vi "LabVIEW Picture.vi"() -> ()   [LabVIEW 2012]
panel:
  out "DeviceIsOpen":bool
  out "Image":T1(plugin-control)
  out "Oil Value":sgl
  out "Water Value":sgl
  out "Output Picture 2":picture
  in  "Temporary File Path 2":path=path "E:/workforpetrol/Tem.bmp"
  in  "TempLate File 2":path=path "E:/workforpetrol/Temp/Template9.png"
  in  "Device Config File Path":path=path "E:/workforpetrol/image device.dat"
  in  "ICImagingControl":refnum<k7>(container)
  in  "Open Device Configuration (Monochrome  Images)":bool
  in  "End Program":bool
  # "Open Device Configuration"
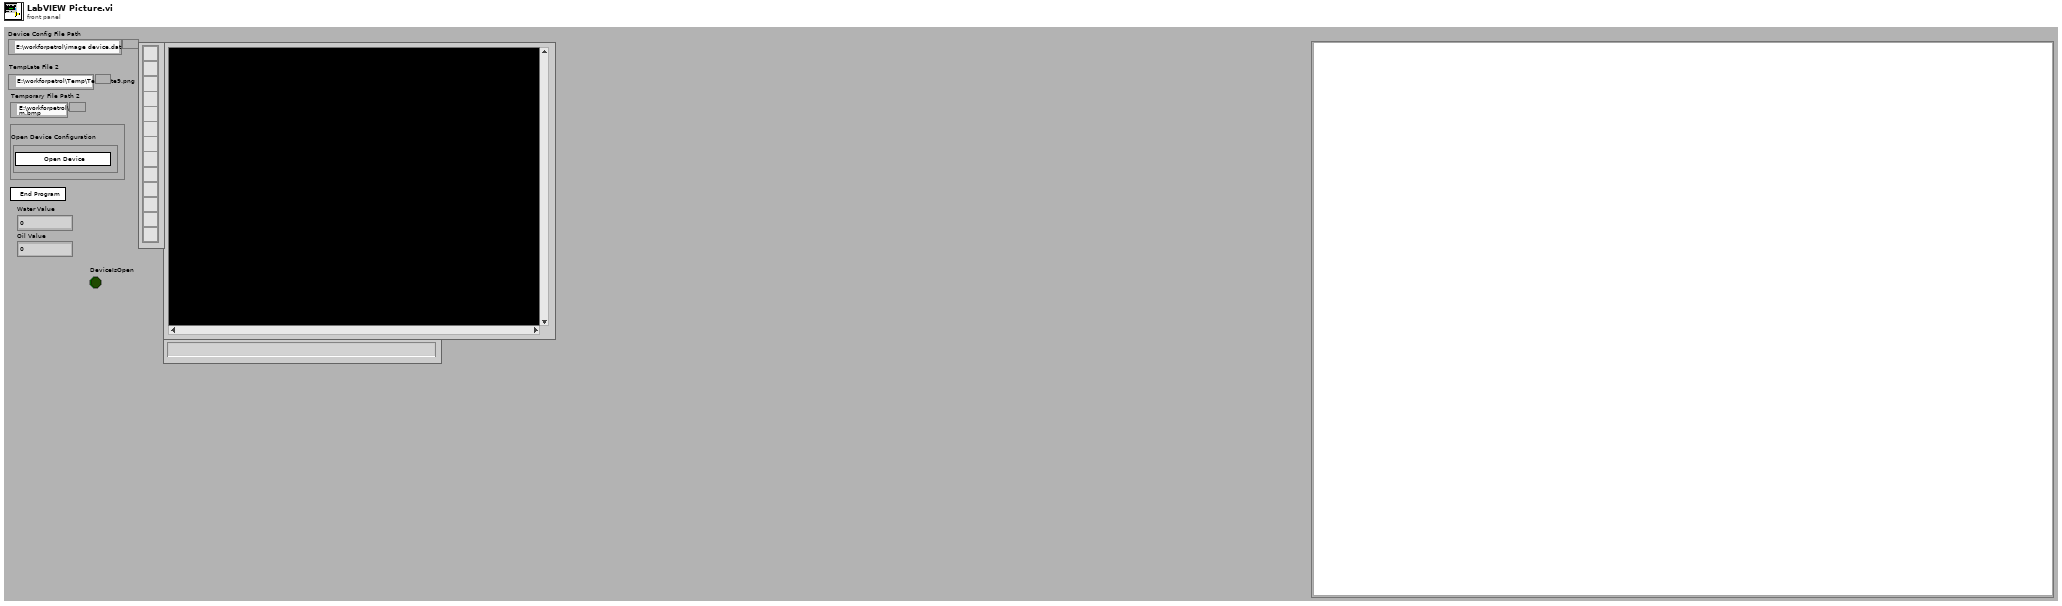
[diagram p1: front panel]
types:
  T1 = typedef "IMAQ Image.ctl" = refnum<image>
  T2 = typedef "imagedata.ctl" = cluster{"image type":i32, "image depth":i32, "image":u8[], "mask":u8[], "colors":u32[], "Rectangle":cluster{"left":i16, "top":i16, "right":i16, "bottom":i16}}
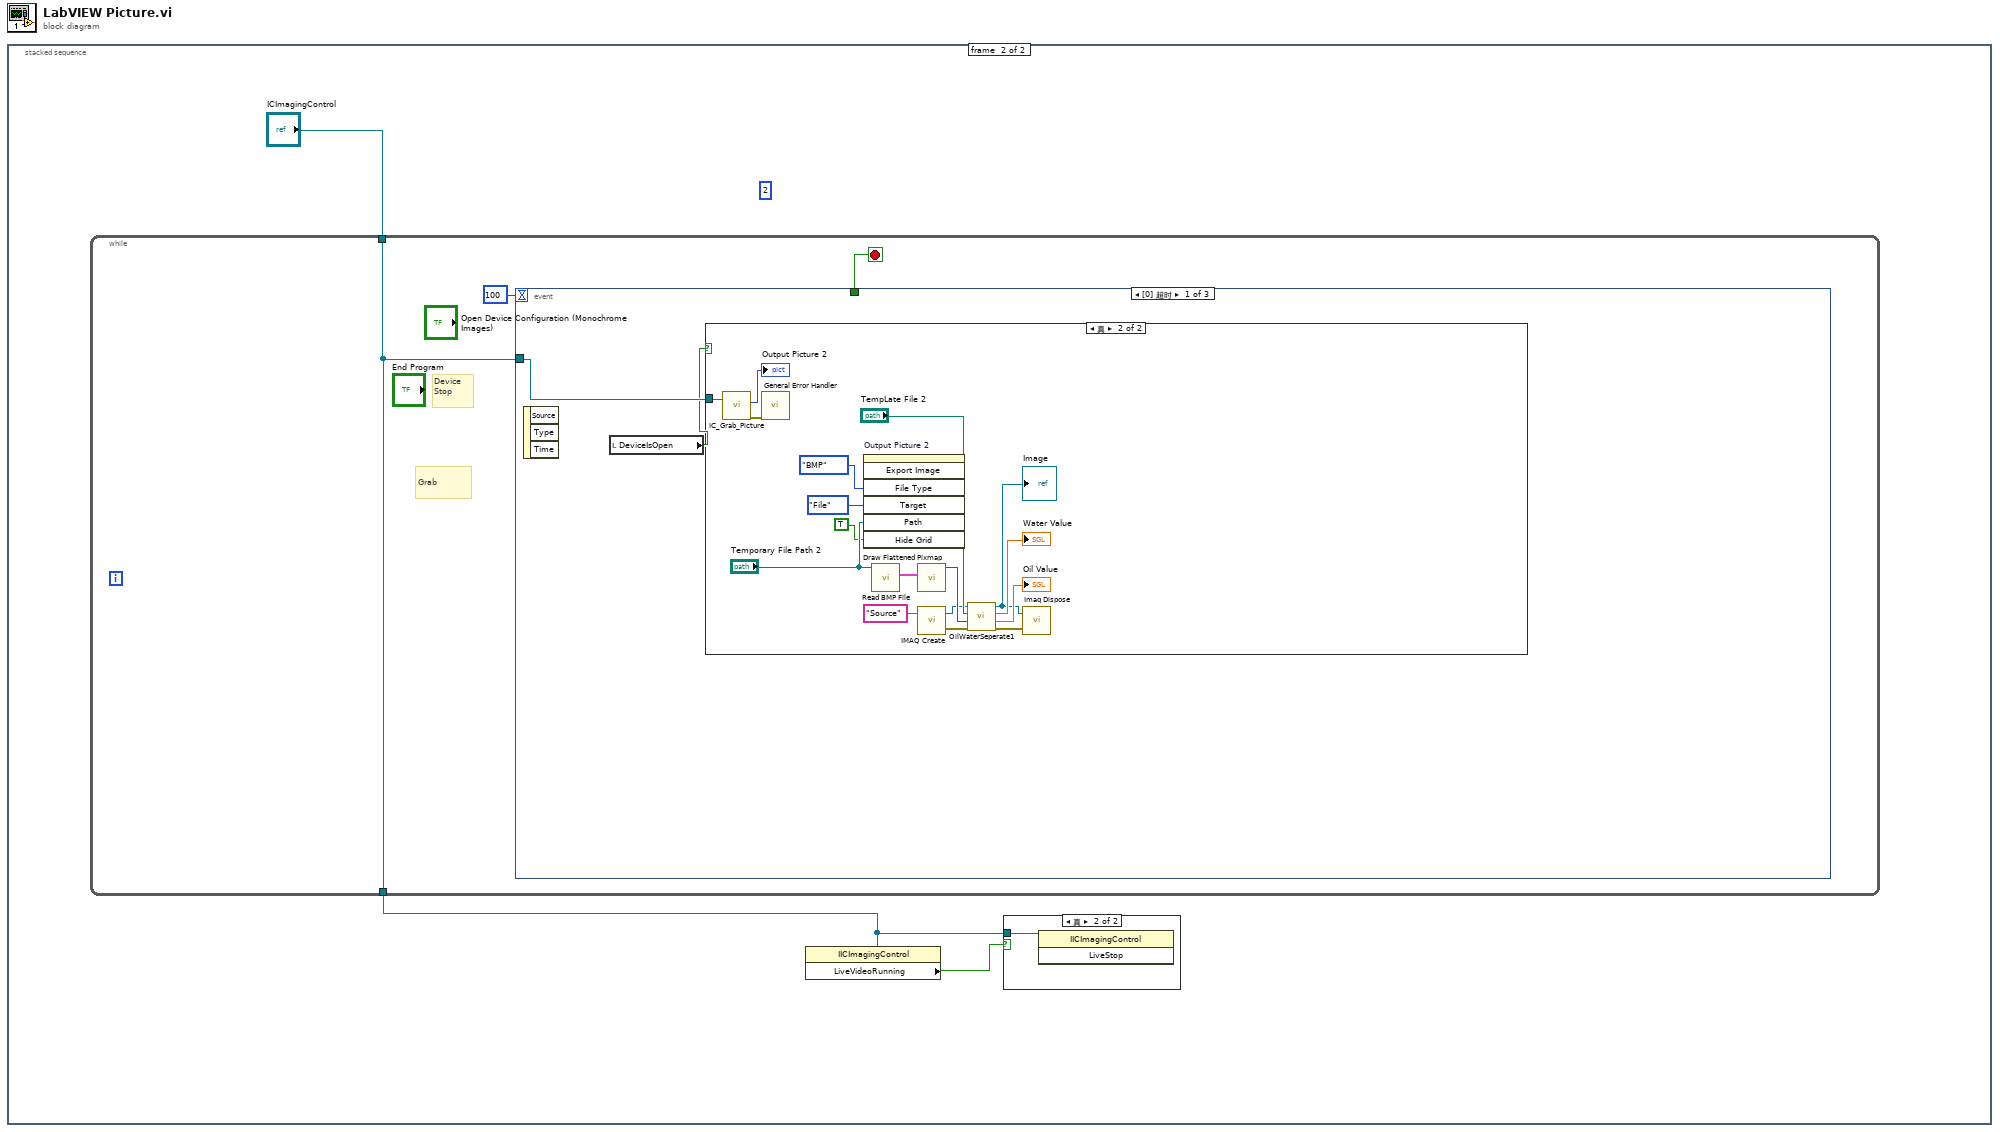
[diagram p0: block diagram]
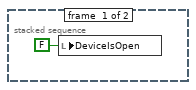
[diagram p2: hidden frame]
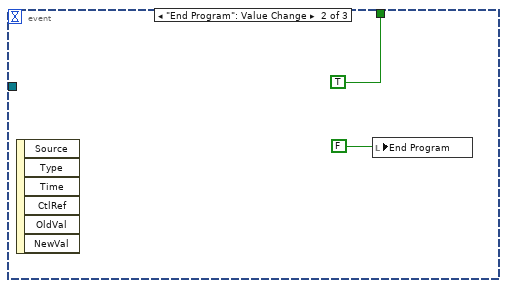
[diagram p5: hidden frame]
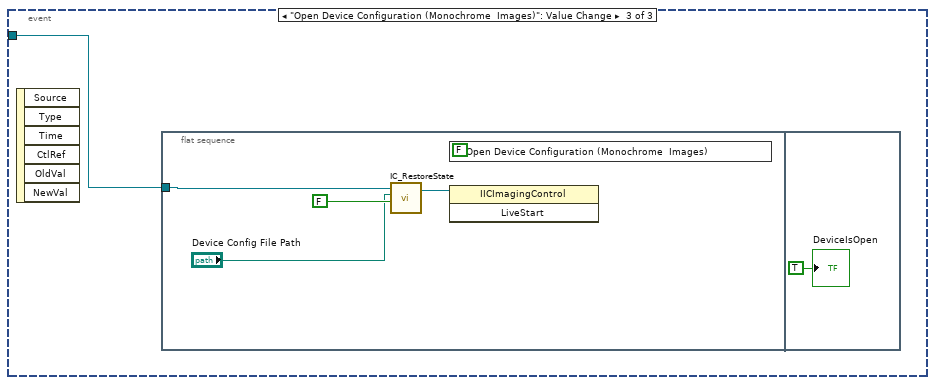
[diagram p6: hidden frame]
diagram:
  n1 = stacked-sequence {
    frame #0 {
      n2 = local write "DeviceIsOpen"(FALSE ("DeviceIsOpen")) -> ()
    }
    frame #1 {
      (unwired) u8 2 ("Disabled")
      n3 = while {
        tunnel: "ICImagingControl" -> [w7]
        tunnel: [w7] -> w3
        stop <- w8 stop-if-true
        # "Device\nStop"
        # "Grab"
        n4 = event shown="[0] 超时" {
          selector: _ -> [_ _ _]
          dyn-events: _ -> [_ _ _]
          timeout: 100 -> [_ _ _]
          tunnel: w7 -> [w10 _ w30]
          tunnel: [_ TRUE _] -> w8
          event Timeout {
            n5 = event-data() -> ()  [unwired: 1 in, 3 out]
            n6 = local read "DeviceIsOpen"() -> (w9:bool)
            n7 = case shown="真" w9 {
              tunnel: w10 -> [_ w25]
              frame False {
              }
              frame True {
                n8 = call "IC_Grab_Picture.vi"("ICImagingControl In"=w25) -> ("Picture Out"=→"Output Picture 2":picture, "Error Out"=w27:errorcluster)  [unwired: 1 in, 2 out]
                n9 = call <vilib>:"General Error Handler.vi"("error in (no error)"=w27) -> ()  [unwired: 10 in, 5 out]
                n10 = invoke on="Output Picture 2" class="Pict" method="Export Image"("File Type"=enum32{"BMP", "EPS", "EMF", "PICT"}."BMP" ("文件类型"), "Target"=enum32{"File", "Clipboard"}."File" ("目标"), "Path"="Temporary File Path 2", "Hide Grid"=TRUE ("始终覆盖")) -> ()  [unwired: 3 in, 7 out]
                n11 = call <vilib>:"Read BMP File.vi"("path to BMP file"="Temporary File Path 2") -> ("image data"=w18:T2)  [unwired: 8 in, 2 out]
                n12 = call <vilib>:"Draw Flattened Pixmap.vi"("image data"=w18) -> ("new picture"=w19:picture)  [unwired: 8 in]
                n13 = call "IMAQ Create"("Image Name"="Source") -> ("New Image"=w12:T1, "error out"=w17:errorcluster)  [unwired: 4 in]
                n14 = call "OilWaterSeperate1.vi"("error in (no error)"=w17, "2D Picture"=w19, "Temp path"="TempLate File 2", "Image in"=w12) -> ("error out"=w20:errorcluster, "Oil Value"=→"Oil Value":sgl, "Water Value"=→"Water Value":sgl, "Image Out"=w11:T1)  [unwired: 4 in]
                "Image" <- w11
                n15 = call "Imaq Dispose"("Image"=w11, "error in (no error)"=w20) -> ()  [unwired: 4 in, 1 out]
              }
            }
          }
          event "End Program": Value Change {
            n16 = event-data() -> ()  [unwired: 1 in, 6 out]
            n17 = local write "End Program"(FALSE) -> ()
          }
          event "Open Device Configuration (Monochrome  Images)": Value Change {
            n18 = event-data() -> ()  [unwired: 1 in, 6 out]
            n19 = flat-sequence {
              tunnel: w30 -> [w33]
              frame #0 {
                n20 = call <userlib>:"IC_RestoreState.vi"("Color"=FALSE, "File Path"="Device Config File Path", "ICImagingControl"=w33) -> ("ICImagingControl Out"=w34:refnum<k7>)  [unwired: 1 in, 1 out]
                n21 = local write "Open Device Configuration (Monochrome  Images)"(FALSE) -> ()
                n22 = invoke class="IICImagingControl" method="LiveStart"(reference=w34) -> ()  [unwired: 2 in, 3 out]
              }
              frame #1 {
                "DeviceIsOpen" <- TRUE ("DeviceIsOpen")
              }
            }
          }
        }
      }
      n23 = property class="IICImagingControl"(reference=w3) -> ("LiveVideoRunning"=w4:bool)  [unwired: 1 in, 2 out]
      n24 = case shown="真" w4 {
        tunnel: w3 -> [_ w5]
        frame False {
        }
        frame True {
          n25 = invoke class="IICImagingControl" method="LiveStop"(reference=w5) -> ()  [unwired: 2 in, 3 out]
        }
      }
    }
  }
